vi "Configure Model.vi"(8 "error in (no error)":errorcluster, 10 "Model in":refnum<class "Model.lvclass">, 11 "Boot Loader in":refnum<class "Boot Loader.lvclass">) -> (0 "error out":errorcluster, 2 "Model out":refnum<class "Model.lvclass">, 3 "Boot Loader out":refnum<class "Boot Loader.lvclass">)   [LabVIEW 2016, in "Boot Loader.lvclass"]
uses:
  Boot Loader.lvclass
  Model/Model.lvclass
  Model/Model.lvclass/Model.ctl
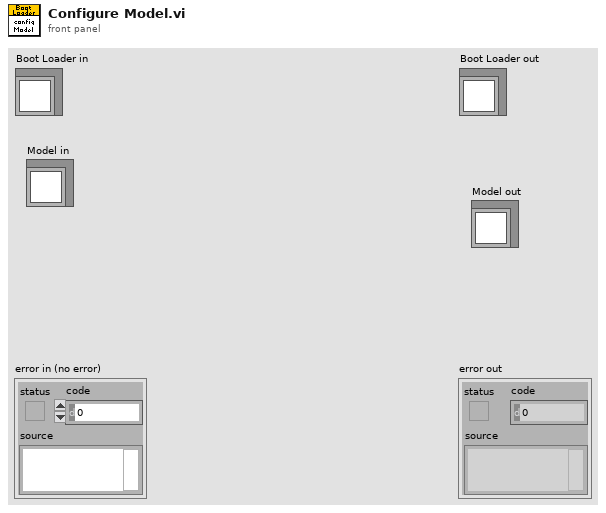
[diagram p1: front panel]
types:
  T1 = typedef "FAMT Typedefs.lvlib/ForceActuatorBoosterValveGainSettings.ctl" = cluster{"AxialBoosterValveGain":sgl, "LateralBoosterValveGain":sgl}
  T2 = typedef "FAMT Typedefs.lvlib/FullForceScanSettings.ctl" = cluster{"Force Tolerance (N)":dbl, "DAA Force Set Points":T3[], "Process Time (s)":dbl, "Sample Time (s)":dbl, "Max Moment (NM)":dbl, "SAA Force Set Points":T3[]}
  T3 = typedef "FAMT Typedefs.lvlib/ForcePair.ctl" = cluster{"Axial Force":dbl, "Lateral Force":dbl}
  T4 = typedef "FAMT Typedefs.lvlib/ForceTableSettings.ctl" = cluster{"Entries":T5[]}
  T5 = typedef "FAMT Typedefs.lvlib/ForceTableEntry.ctl" = cluster{"ID":string, "Force Set Points":T3[]}
  T6 = typedef "FAMT Typedefs.lvlib/OperationalForceTestSettings.ctl" = cluster{"Max Force Error (N)":dbl, "Max Moment (NM)":dbl, "Process Time (s)":dbl, "Sample Time (s)":dbl}
  T7 = typedef "FAMT Typedefs.lvlib/DifferentialPressureReleaseValveTestSettings.ctl" = cluster{"Max Over Force (N)":dbl, "Max Moment (NM)":dbl, "Process Time (s)":dbl, "Sample Time (s)":dbl}
  T8 = typedef "FAMT Typedefs.lvlib/ForceAccuracyTestSettings.ctl" = cluster{"Max Force Error (N)":dbl, "Max Moment (NM)":dbl, "Process Time (s)":dbl, "Sample Time (s)":dbl, "Iterations":i32, "Amplitude (N)":dbl, "Non-Repeating Error":dbl}
  T9 = typedef "FAMT Typedefs.lvlib/SentranAccuracyTestSettings.ctl" = cluster{"Force Tolerance (N)":dbl, "Force Modifies (%)":dbl[], "Process Time (s)":dbl, "Sample Time (s)":dbl, "Max Moment (NM)":dbl}
  T10 = typedef "FAMT Typedefs.lvlib/TrackingTestSettings.ctl" = cluster{"Max Force Error (N)":dbl, "Max Moment (NM)":dbl, "Process Time (s)":dbl, "Sample Time (s)":dbl, "Iterations":i32, "Amplitude (N)":dbl, "Non-Repeating Error":dbl}
  T11 = typedef "FAMT Typedefs.lvlib/SlewingTestSettings.ctl" = cluster{"Max Force Error (N)":dbl, "Max Moment (NM)":dbl, "Amplitude (N)":dbl, "Max Instance Force Error (N)":dbl, "Ramp Time (s)":dbl, "Hold Time (s)":dbl, "Settling Time (s)":dbl}
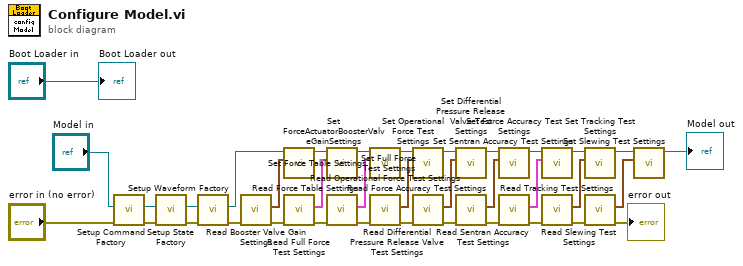
[diagram p0: block diagram]
diagram:
  n1 = call "Setup Command Factory.vi"("error in (no error)"="error in (no error)", "Model in"="Model in") -> ("error out"=w33:errorcluster, "Model out"=w35:refnum<class "Model.lvclass">)  [unwired: 7 in, 1 out]
  n2 = call "Setup State Factory.vi"("error in (no error)"=w33, "Model in"=w35) -> ("error out"=w32:errorcluster, "Model out"=w34:refnum<class "Model.lvclass">)  [unwired: 7 in, 1 out]
  n3 = call "Setup Waveform Factory.vi"("error in (no error)"=w32, "Model in"=w34) -> ("error out"=w5:errorcluster, "Model out"=w2:refnum<class "Model.lvclass">)  [unwired: 7 in, 1 out]
  n4 = call "Read Booster Valve Gain Settings.vi"("error in (no error)"=w5) -> ("error out"=w4:errorcluster, "ForceActuatorBoosterValveGainSettings"=w3:T1)  [unwired: 8 in, 1 out]
  n5 = call "Set ForceActuatorBoosterValveGainSettings.vi"("ForceActuatorBoosterValveGainSettings"=w3, "Model in"=w2) -> ("Model out"=w1:refnum<class "Model.lvclass">)  [unwired: 9 in]
  n6 = call "Read Full Force Test Settings.vi"("error in (no error)"=w4) -> ("error out"=w29:errorcluster, "Full Force Test Settings"=w30:T2)  [unwired: 8 in, 1 out]
  n7 = call "Set Full Force Test Settings.vi"("Full Force Test Settings"=w30, "Model in"=w1) -> ("Model out"=w28:refnum<class "Model.lvclass">)  [unwired: 9 in]
  n8 = call "Read Force Table Settings.vi"("error in (no error)"=w29) -> ("error out"=w25:errorcluster, "Force Table Settings"=w27:T4)  [unwired: 8 in, 1 out]
  n9 = call-dynamic "Set Force Table Settings.vi"("Force Table Settings"=w27, "Model in"=w28) -> ("Model out"=w26:refnum<class "Model.lvclass">)  [unwired: 9 in]
  n10 = call "Read Operational Force Test Settings.vi"("error in (no error)"=w25) -> ("error out"=w23:errorcluster, "Operational Force Test Settings"=w24:T6)  [unwired: 8 in, 1 out]
  n11 = call-dynamic "Set Operational Force Test Settings.vi"("Operational Force Test Settings"=w24, "Model in"=w26) -> ("Model out"=w22:refnum<class "Model.lvclass">)  [unwired: 9 in]
  n12 = call "Read Differential Pressure Release Valve Test Settings.vi"("error in (no error)"=w23) -> ("error out"=w20:errorcluster, "Differential Pressure Release Valve Test Settings"=w21:T7)  [unwired: 8 in, 1 out]
  n13 = call-dynamic "Set Differential Pressure Release Valve Test Settings.vi"("Differential Pressure Release Valve Test Settings"=w21, "Model in"=w22) -> ("Model out"=w19:refnum<class "Model.lvclass">)  [unwired: 9 in]
  n14 = call "Read Force Accuracy Test Settings.vi"("error in (no error)"=w20) -> ("error out"=w17:errorcluster, "Force Accuracy Test Settings"=w18:T8)  [unwired: 8 in, 1 out]
  n15 = call-dynamic "Set Force Accuracy Test Settings.vi"("Force Accuracy Test Settings"=w18, "Model in"=w19) -> ("Model out"=w15:refnum<class "Model.lvclass">)  [unwired: 9 in]
  n16 = call "Read Sentran Accuracy Test Settings.vi"("error in (no error)"=w17) -> ("error out"=w12:errorcluster, "Sentran Accuracy Test Settings"=w16:T9)  [unwired: 8 in, 1 out]
  n17 = call "Set Sentran Accuracy Test Settings.vi"("Sentran Accuracy Test Settings"=w16, "Model in"=w15) -> ("Model out"=w13:refnum<class "Model.lvclass">)  [unwired: 9 in]
  n18 = call "Read Tracking Test Settings.vi"("error in (no error)"=w12) -> ("error out"=w11:errorcluster, "Tracking Test Settings"=w14:T10)  [unwired: 8 in, 1 out]
  n19 = call "Set Tracking Test Settings.vi"("Tracking Test Settings"=w14, "Model in"=w13) -> ("Model out"=w10:refnum<class "Model.lvclass">)  [unwired: 9 in]
  n20 = call "Read Slewing Test Settings.vi"("error in (no error)"=w11) -> ("error out"=→"error out":errorcluster, "Slewing Test Settings"=w9:T11)  [unwired: 8 in, 1 out]
  n21 = call "Set Slewing Test Settings.vi"("Slewing Test Settings"=w9, "Model in"=w10) -> ("Model out"=→"Model out":refnum<class "Model.lvclass">)  [unwired: 9 in]
  "Boot Loader out" <- "Boot Loader in"
